vi "clean_up_instruments (SubVI).vi"(11 "instrum out":T1) -> ()   [LabVIEW 2014]
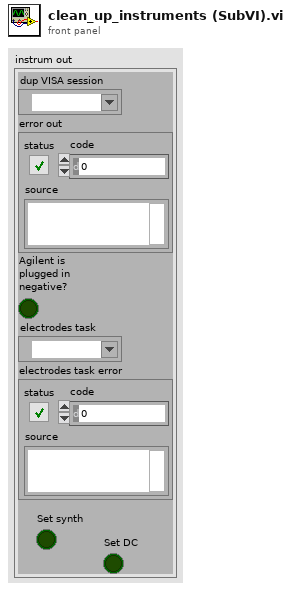
[diagram p1: front panel]
types:
  T1 = cluster{"dup VISA session":refnum<visa-resource-name>, "error out":errorcluster, "Agilent is \nplugged in \nnegative?":bool, "electrodes task":refnum<k21>, "electrodes task error":errorcluster, "Set synth":bool, "Set DC":bool}
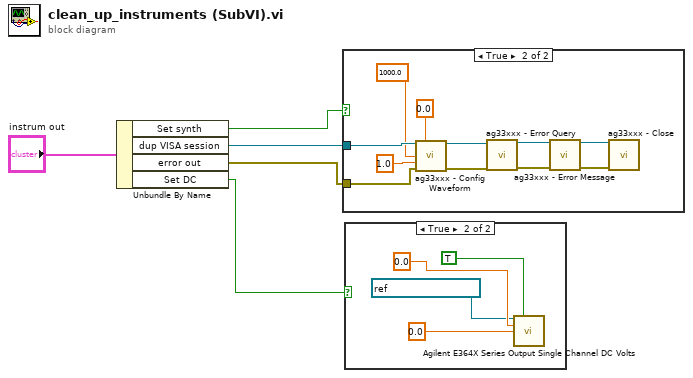
[diagram p0: block diagram]
diagram:
  n1 = Unbundle By Name("instrum out") -> ("Set synth"=w4:bool, "dup VISA session"=w3:refnum<visa-resource-name>, "error out"=w2:errorcluster, "Set DC"=w1:bool)
  n2 = case shown="True" w4 {
    tunnel: w2 -> [_ w16]
    tunnel: w3 -> [_ w15]
    frame False {
    }
    frame True {
      n3 = call "ag33xxx - Config Waveform.vi"("VISA session"=w15, "Offset (0.00 V)"=0.0, "Frequency (1000 Hz)"=1000.0, "Amplitude (0.1 Vpp)"=1.0, "error in (no error)"=w16) -> ("dup VISA session"=w8:refnum<visa-resource-name>, "error out"=w10:errorcluster)  [unwired: 9 in]
      n4 = call "ag33xxx - Error Query.vi"("error in (no error)"=w10, "VISA session"=w8) -> ("error out"=w11:errorcluster, "dup VISA session"=w12:refnum<visa-resource-name>)  [unwired: 6 in, 2 out]
      n5 = call "ag33xxx - Error Message.vi"("VISA session"=w12, "error in (no error)"=w11) -> ("dup VISA session"=w7:refnum<visa-resource-name>, "error out"=w9:errorcluster)  [unwired: 9 in, 3 out]
      n6 = call "ag33xxx - Close.vi"("error in (no error)"=w9, "VISA session"=w7) -> ()  [unwired: 9 in, 1 out]
    }
  }
  n7 = case shown="True" w1 {
    frame False {
    }
    frame True {
      n8 = call <instrlib>:"Agilent E364X Series Output Single Channel DC Volts.vi"("VISA resource name"=refnum<visa-resource-name> "GPIB0::8::INSTR", "Output Enabled (False)"=TRUE, "Voltage Level (0.0 Volts)"=0.0, "Current Limit (0 Amps)"=0.0) -> ()  [unwired: 11 in, 1 out]
    }
  }
